vi "Actor Core.vi"(8 "error in":errorcluster, 11 "Chronometer in":refnum<class "Chronometer.lvclass">) -> (0 "error out":errorcluster, 3 "Actor out":refnum<class "Actor.lvclass">)   [LabVIEW 2023, in "Chronometer.lvlib" / "Chronometer.lvclass"]
doc: "The user interface for this panel.\n\n----\nPlease see the following web address for additional documentation and tutorial information:\nhttp://www.mooregoodideas.com/mgi-panel-manager/\n\nAuthor: Derek Trepanier\n\nCopyright (c) 2018, Moore Good Ideas, Inc.\n\nAll rights reserved.\n\nRedistribution and use in source and binary forms, with or without modification, are permitted provided that the following conditions are met:\n\n * Redistributions of source code must retain the above copyright notice, this list of conditions and the following disclaimer.\n * Redistributions in binary form must reproduce the above copyright notice, this list of conditions and the following disclaimer in the documentation and/or other materials provided with the distribution.\n * Neither the name of Moore Good Ideas, Inc. nor the names of its contributors may be used to endorse or promote products derived from this software without specific prior written permission.\n\nTHIS SOFTWARE IS PROVIDED BY THE COPYRIGHT HOLDERS AND CONTRIBUTORS \"AS IS\" AND ANY EXPRESS OR IMPLIED WARRANTIES, INCLUDING, BUT NOT LIMITED TO, THE IMPLIED WARRANTIES OF MERCHANTABILITY AND FITNESS FOR A PARTICULAR PURPOSE ARE DISCLAIMED. IN NO EVENT SHALL THE COPYRIGHT OWNER OR CONTRIBUTORS BE LIABLE FOR ANY DIRECT, INDIRECT, INCIDENTAL, SPECIAL, EXEMPLARY, OR CONSEQUENTIAL DAMAGES (INCLUDING, BUT NOT LIMITED TO, PROCUREMENT OF SUBSTITUTE GOODS OR SERVICES; LOSS OF USE, DATA, OR PROFITS; OR BUSINESS INTERRUPTION) HOWEVER CAUSED AND ON ANY THEORY OF LIABILITY, WHETHER IN CONTRACT, STRICT LIABILITY, OR TORT (INCLUDING NEGLIGENCE OR OTHERWISE) ARISING IN ANY WAY OUT OF THE USE OF THIS SOFTWARE, EVEN IF ADVISED OF THE POSSIBILITY OF SUCH DAMAGE."
uses:
  Chronometer.lvclass
  C:/Users/Public/Documents/Development/builds/Engine/Engine.lvlibp/Project/Engine.lvclass
  builds/Engine/Actor Framework.lvlibp/1abvi3w/vi.lib/ActorFramework/Actor/Actor.lvclass
  Chronometer Messages/Set UUT Supply State Msg/Set UUT Supply State Msg.lvclass/Set UUT Supply State Msg.ctl
  builds/Engine/Engine.lvlibp/Accessors/Read Self Q.vi
  builds/Engine/Actor Framework.lvlibp/1abvi3w/vi.lib/ActorFramework/Message Enqueuer/Enqueue.vi
  builds/Engine/Actor Framework.lvlibp/1abvi3w/vi.lib/ActorFramework/Message Enqueuer/Message Enqueuer.lvclass
  Chronometer Messages/Set UUT Supply State Msg/Set UUT Supply State Msg.lvclass
  builds/Tools/Config.lvlibp/Config.lvclass
types:
  T1 = cluster{"Pnl Actor":refnum<event-registration>, "Event Registration Refnum":refnum<event-registration>}
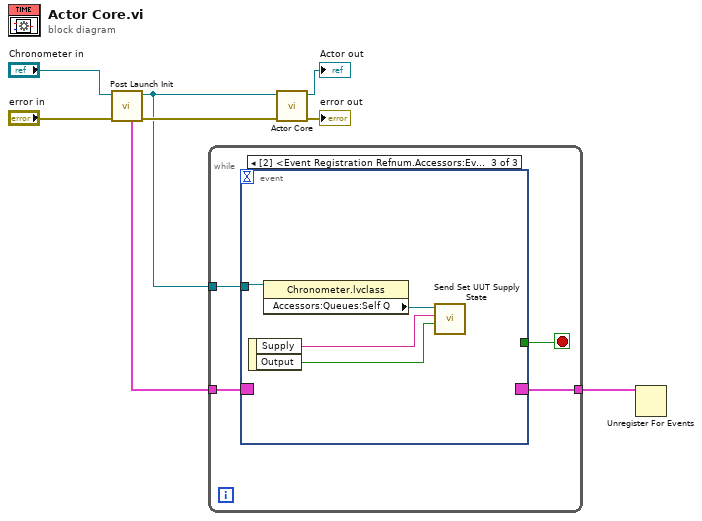
[diagram p0: block diagram]
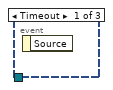
[diagram p2: hidden frame]
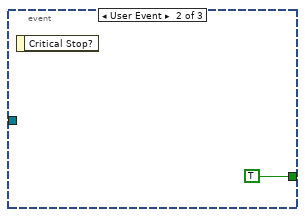
[diagram p3: hidden frame]
diagram:
  n1 = call "Post Launch Init.vi"("error in"="error in", "Chronometer in"="Chronometer in") -> ("error out"=w5:errorcluster, "Chronometer out"=w1:refnum<class "Chronometer.lvclass">, "Events"=w3:T1)  [unwired: 7 in]
  n2 = while {
    tunnel: w3 -> [w12]
    tunnel: [w10] -> w2
    tunnel: w1 -> [w9]
    stop <- w11 stop-if-true
    n3 = event shown="[2] <Event Registration Refnum.Accessors:Events:All.Manual.UUTSupply>: User Event" {
      selector: w12 -> [_ _ _]
      dyn-events: [_ _ _] -> w10
      timeout: _ -> [_ _ _]
      tunnel: [_ TRUE _] -> w11
      tunnel: w9 -> [_ _ w17]
      event Timeout {
        n4 = event-data() -> ()  [unwired: 1 in, 1 out]
      }
      event User Event {
        n5 = event-data() -> ()  [unwired: 1 in, 1 out]
      }
      event User Event {
        n6 = event-data() -> ("Supply"=w15:string, "Output"=w14:bool)  [unwired: 1 in]
        n7 = property class="Chronometer.lvclass"(reference=w17) -> ("Accessors:Queues:Self Q"=w16:refnum<class "Message Enqueuer.lvclass">)  [unwired: 1 in, 2 out]
        n8 = call "Send Set UUT Supply State.vi"("Output"=w14, "Supply_ID"=w15, "Message Enqueuer"=w16) -> ()  [unwired: 7 in, 2 out]
      }
    }
  }
  n9 = call-parent "Actor Core.vi"("error in"=w5, "State Actor in"=w1) -> ("error out"=→"error out":errorcluster, "Actor out"=→"Actor out":refnum<class "Actor.lvclass">)  [unwired: 8 in]
  n10 = Unregister For Events(event registration refnum=w2) -> ()  [unwired: 1 in, 1 out]
